vi "Pre Build.vi"(0 "VIP in":refnum<class "VIP.lvclass">) -> (4 "VIP out":refnum<class "VIP.lvclass">)   [LabVIEW 2017, in "CL_G3_VIComponentBuilder.lvlib" / "VIP.lvclass"]
doc: "Runs the pre install steps for the vi package. This ensures that the components needed dependencies (like vendor drivers) are installed."
uses:
  VIP.lvclass
  C:/builds/Component BuilderBT/SrcDist/Exports/Exports/Export.lvclass
  Exports/Export.lvclass/Export.ctl
  Exports/Accessors/Read Export Build Specification.vi
  Exports/Accessors/Write Export Operation Errors.vi
  Exports/Accessors/Read Export Operation Errors.vi
  Exports/Export.lvclass
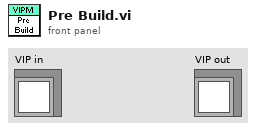
[diagram p1: front panel]
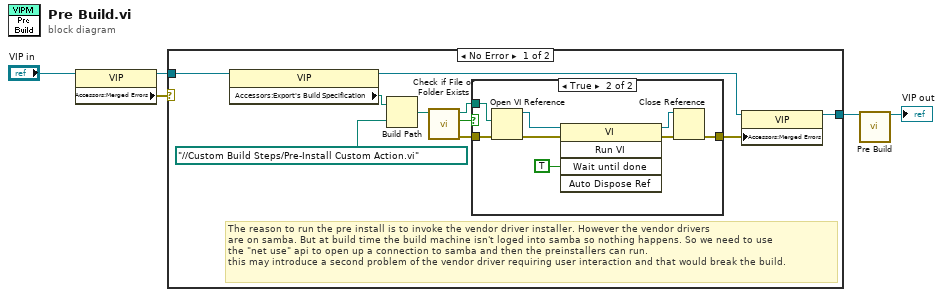
[diagram p0: block diagram]
diagram:
  n1 = property class="VIP"(reference="VIP in") -> (reference out=w1:refnum<class "VIP.lvclass">, "Accessors:Merged Errors"=w2:errorcluster)  [unwired: 1 in, 1 out]
  n2 = case shown="No Error" w2 {
    tunnel: w1 -> [w11 w25]
    tunnel: [w6 w25] -> w5
    frame No Error {
      # "The reason to run the pre install is to invoke the vendor driver installer. However the vendor drivers\nare on samba. But at build time the build machine isn't loged into samba so nothing happens. So we need to use\nthe \"net use\" api to open up a connection to samba and then the preinstallers can run. \nthis may introduce a second problem of the vendor driver requiring user interaction and that would break the build."
      n3 = property class="VIP"(reference=w11) -> (reference out=w10:refnum<class "VIP.lvclass">, "Accessors:Export's Build Specification"=w9:path)  [unwired: 1 in, 1 out]
      n4 = Build Path(base path=w9, name or relative path=path "../../Custom Build Steps/Pre-Install Custom Action.vi" ("path")) -> (appended path=w13:path)
      n5 = call <vilib>:"Check if File or Folder Exists.vi"("path"=w13) -> ("error out"=w8:errorcluster, "file or folder exists?"=w14:bool, "dup path"=w15:path)  [unwired: 8 in]
      n6 = case shown="True" w14 {
        tunnel: w15 -> [_ w24]
        tunnel: w8 -> [w16 w18]
        tunnel: [w16 w17] -> w7
        frame False {
        }
        frame True {
          n7 = Open VI Reference(vi path=w24, error in (no error)=w18) -> (vi reference=w23:refnum<vi>, error out=w20:errorcluster)  [unwired: 4 in]
          n8 = invoke class="VI" method="Run VI"(reference=w23, error in=w20, "Wait until done"=TRUE ("Wait Until Done")) -> (reference out=w21:refnum<vi>, error out=w22:errorcluster)  [unwired: 2 in, 3 out]
          n9 = Close Reference(reference=w21, error in (no error)=w22) -> (error out=w17:errorcluster)
        }
      }
      n10 = property class="VIP"(reference=w10, "Accessors:Merged Errors"=w7) -> (reference out=w6:refnum<class "VIP.lvclass">)  [unwired: 1 in, 1 out]
    }
    frame Error {
    }
  }
  n11 = call-parent "Pre Build.vi"("Export In"=w5) -> ("Export out"=→"VIP out":refnum<class "VIP.lvclass">)  [unwired: 14 in]
